vi "Available GPIO.vi"(8 "error in (no error)":errorcluster, 11 "VisaComms in":refnum<class "VisaComms.lvclass">) -> (0 "error out":errorcluster, 2 "Available GPIO":T1[](array[typedef]), 3 "VisaComms out":refnum<class "VisaComms.lvclass">)   [LabVIEW 2024, in "CTI.lvlib" / "VisaComms.lvclass"]
uses:
  VisaComms.lvclass
  GPIO Number.ctl
  VisaComms.lvclass/VisaComms.ctl
  Clean Visa Errors.vi
  CTI.lvlib
panel:
  out "Buffer":string
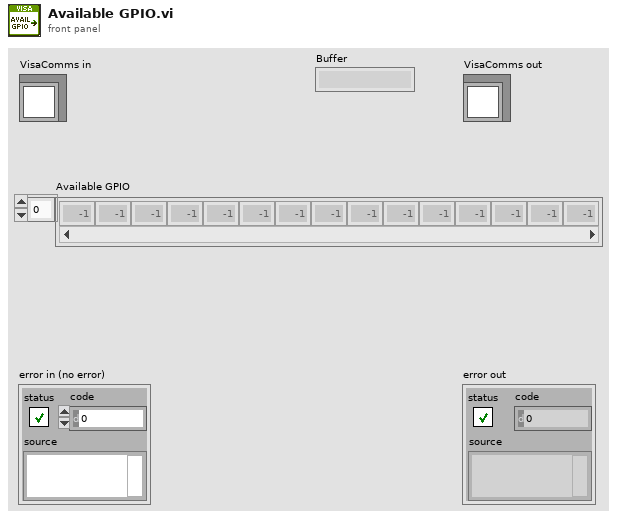
[diagram p1: front panel]
types:
  T1 = typedef "CTI.lvlib/GPIO Number.ctl" = i8
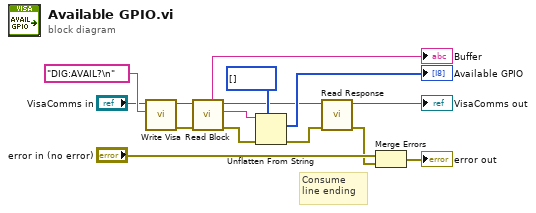
[diagram p0: block diagram]
diagram:
  # "Consume line ending"
  n1 = call "Write Visa.vi"("write buffer"="DIG:AVAIL?\n", "VisaComms in"="VisaComms in") -> ("error out"=w12:errorcluster, "VisaComms out"=w13:refnum<class "VisaComms.lvclass">)  [unwired: 7 in, 1 out]
  n2 = call "Read Block.vi"("error in (no error)"=w12, "VisaComms in"=w13) -> ("error out"=w15:errorcluster, "Block"=w11:string, "VisaComms out"=w2:refnum<class "VisaComms.lvclass">, "Buffer"=→"Buffer":string)  [unwired: 6 in]
  n3 = Unflatten From String(type=T1[] [] ("Available GPIO"), binary string=w11, error in (no error)=w15) -> (value=→"Available GPIO":T1[], error out=w10:errorcluster)  [unwired: 2 in, 1 out]
  n4 = call "Read Response.vi"("error in (no error)"=w10, "VisaComms in"=w2) -> ("error out"=w3:errorcluster, "VisaComms out"=→"VisaComms out":refnum<class "VisaComms.lvclass">)  [unwired: 6 in, 2 out]
  n5 = Merge Errors("error in (no error)", w3) -> (→"error out":errorcluster)
